vi "Fmt_MsgToService.vi"(10 "Data":string, 11 "state":string) -> (3 "<JSON>":string)   [LabVIEW 2020]
uses:
  0dad44f8-3da4-4488-a1cb-9186d07aba80.vi
  <vilib>/JDP Science/JSONtext/JSONtext.lvlib
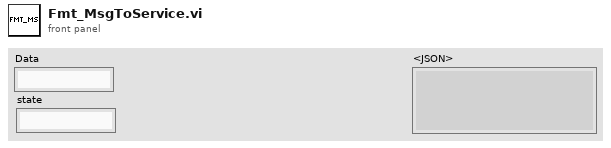
[diagram p1: front panel]
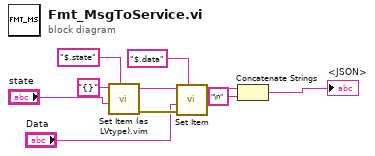
[diagram p0: block diagram]
diagram:
  n1 = call "Set Item (as LVtype).vim"("Object (or Item) Path"="$.state", "Anything"="state", "JSON"="{}") -> ("error out"=w5:errorcluster, "<JSON>"=w7:string)  [unwired: 5 in, 1 out]
  n2 = call <vilib>:"Set Item.vi"("$Path or Item Name"="$.data", "error in (no error)"=w5, "JSON to Insert"="Data", "JSON"=w7) -> ("<JSON>"=w3:string)  [unwired: 4 in, 2 out]
  n3 = Concatenate Strings(w3, "\n" ("string")) -> (→"<JSON>":string)
